vi "getRangeAndEnabled.vi"(6 "Enable":bool, 7 "mode":enum16{"enable Channel", "get/set Range"}(ring)=enum."get/set Range", 8 "error in (no error)":errorcluster, 9 "Channel (0.1.2.3)":string="0", 10 "range (V)":dbl, 11 "Refnum in":refnum<k21>) -> (0 "error out":errorcluster, 1 "Enabled (array)":bool[](array[boolean])=[FALSE, TRUE, TRUE, TRUE], 2 "Range":dbl[](array[numeric]), 3 "Refnum out":refnum<k21>)   [LabVIEW 2011]
uses:
  C:/Program Files/National Instruments/LabVIEW 2011/resource/objmgr/daqmx.rc
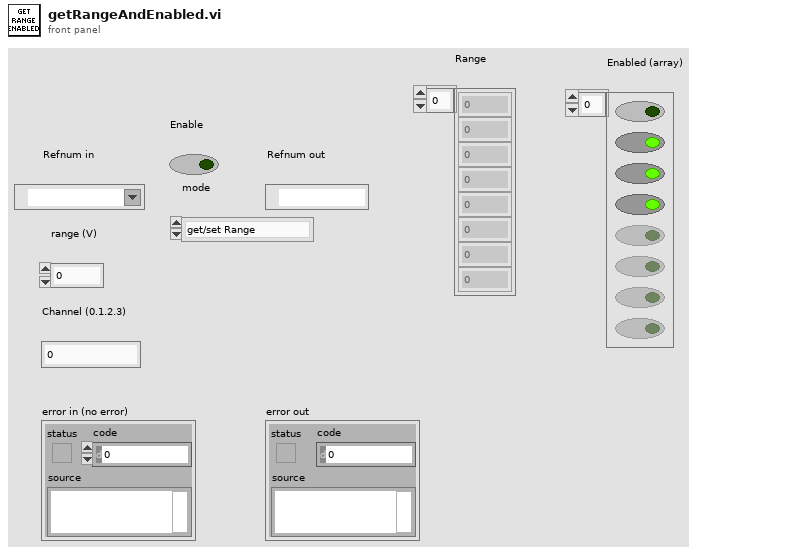
[diagram p1: front panel]
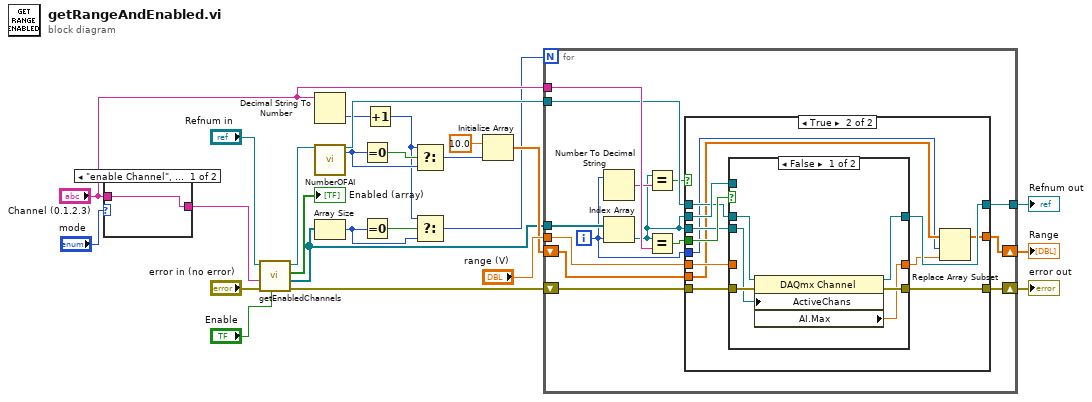
[diagram p0: block diagram]
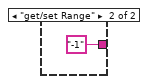
[diagram p2: hidden frame]
diagram:
  n1 = case shown="\"enable Channel\", Default" "mode" {
    tunnel: [w26 "-1" ("Channel (0.1.2.3)")] -> w22
    tunnel: "Channel (0.1.2.3)" -> [w26 _]
    frame "enable Channel", Default {
    }
    frame "get/set Range" {
    }
  }
  n2 = call "getEnabledChannels.vi"("Enable"="Enable", "error in (no error)"="error in (no error)", "Channel (0.1.2.3)"=w22, "Refnum in"="Refnum in") -> ("error out"=w21:errorcluster, "Channels"=w5:refnum<k21>[], "Enable (Array)"=→"Enabled (array)":bool[], "Refnum out"=w14:refnum<k21>)  [unwired: 4 in]
  n3 = Decimal String To Number(string="Channel (0.1.2.3)") -> (number=w9:i32)  [unwired: 2 in, 1 out]
  n4 = call "NumberOFAI.vi"("Refnum in"=w14) -> ("Refnum out"=w13:refnum<k21>, "Numeric"=w7:i32)  [unwired: 16 in, 1 out]
  n5 = Array Size(array=w5) -> (size(s)=w2:i32)
  n6 = Equal To 0?(x=w7) -> (x = 0?=w8:bool)
  n7 = Equal To 0?(x=w2) -> (x = 0?=w4:bool)
  n8 = Increment(x=w9) -> (x+1=w3:i32)
  n9 = Select(t=w3, s=w8, f=w7) -> (s? t:f=w6:i32)
  n10 = Select(t=w3, s=w4, f=w2) -> (s? t:f=w1:i32)
  n11 = Initialize Array(10.0 ("element"), w6) -> (w12:dbl[])
  n12 = for {
    N: w1 -> [_]
    tunnel: "Channel (0.1.2.3)" -> [w41]
    tunnel: "range (V)" -> [w39]
    tunnel: w13 -> [w38]
    tunnel: [w37] -> w16
    shift-right: [w35] -> w25
    shift-left: w21 -> [w36]
    tunnel: w5 -> [w30]
    shift-right: [w31] -> w11
    shift-left: w12 -> [w32]
    i -> [w28]
    n13 = Number To Decimal String(number=w28) -> (decimal integer string=w34:string)  [unwired: 1 in]
    n14 = Index Array(array=w30, index=w28) -> (element=w29:refnum<k21>)
    n15 = Equal?(x=w29, y=w34) -> (x = y?=w33:bool)
    n16 = Equal?(x=w29, y=w41) -> (x = y?=w40:bool)
    n17 = case shown="True" w33 {
      tunnel: w29 -> [_ w56]
      tunnel: w40 -> [_ w55]
      tunnel: w39 -> [_ w54]
      tunnel: w38 -> [w44 w53]
      tunnel: [w44 w52] -> w37
      tunnel: w36 -> [w43 w51]
      tunnel: [w43 w50] -> w35
      tunnel: w29 -> [_ w49]
      tunnel: w32 -> [w42 w48]
      tunnel: [w42 w47] -> w31
      tunnel: w28 -> [_ w46]
      frame False {
      }
      frame True {
        n18 = case shown="False" w55 {
          tunnel: w56 -> [_ _]
          tunnel: [w58 w65] -> w45
          tunnel: w54 -> [_ w65]
          tunnel: w53 -> [w62 w64]
          tunnel: [w61 w64] -> w52
          tunnel: w51 -> [w60 w63]
          tunnel: [w59 w63] -> w50
          tunnel: w49 -> [w57 _]
          frame False {
            n19 = property class="DAQmx Channel"(reference=w62, error in=w60, "ActiveChans"=w57) -> (reference out=w61:refnum<k21>, error out=w59:errorcluster, "AI.Max"=w58:dbl)
          }
          frame True {
          }
        }
        n20 = Replace Array Subset(array=w48, new element=w45, index=w46) -> (w47:dbl[])
      }
    }
  }
  "error out" <- w25
  "Refnum out" <- w16
  "Range" <- w11
